vi "UDP Send (1).vi"(0 "Numeric 7":dbl, 1 "Numeric 3":dbl, 2 "Numeric 2":dbl, 3 "Numeric 4":dbl, 4 "Numeric 9":dbl, 5 "Numeric 8":dbl, 6 "Numeric":dbl, 7 "Numeric 5":dbl, 8 "Numeric 6":dbl) -> ()   [LabVIEW 2012]
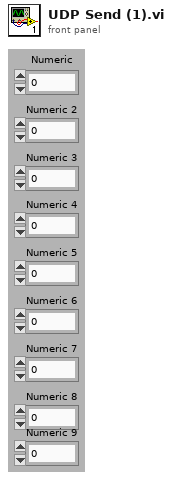
[diagram p1: front panel]
types:
  T1 = cluster{"Numeric":dbl, "Numeric 2":dbl, "Numeric 3":dbl, "Numeric 4":dbl, "Numeric 5":dbl, "Numeric 6":dbl, "Numeric 7":dbl, "Numeric 8":dbl, "Numeric 9":dbl}
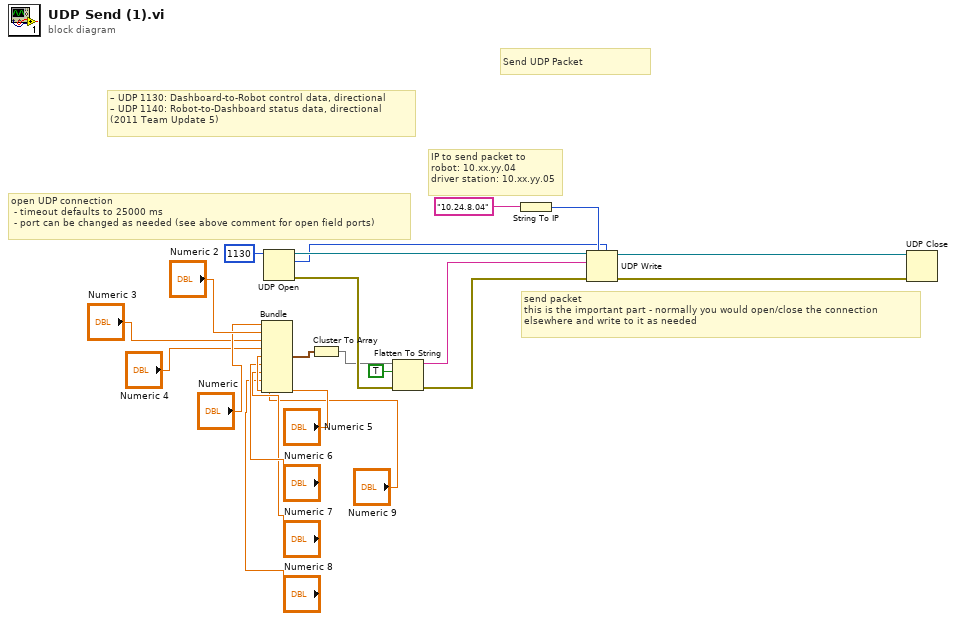
[diagram p0: block diagram]
diagram:
  # "send packet\nthis is the important part - normally you would open/close the connection \nelsewhere and write to it as needed"
  # "IP to send packet to \nrobot: 10.xx.yy.04\ndriver station: 10.xx.yy.05"
  # "open UDP connection\n - timeout defaults to 25000 ms\n - port can be changed as needed (see above comment for open field ports)"
  # "Send UDP Packet"
  # "– UDP 1130: Dashboard-to-Robot control data, directional\n– UDP 1140: Robot-to-Dashboard status data, directional\n(2011 Team Update 5)"
  n1 = Bundle("Numeric"="Numeric", "Numeric 2"="Numeric 2", "Numeric 3"="Numeric 3", "Numeric 4"="Numeric 4", "Numeric 5"="Numeric 5", "Numeric 6"="Numeric 6", "Numeric 7"="Numeric 7", "Numeric 8"="Numeric 8", "Numeric 9"="Numeric 9") -> (w3:T1)  [unwired: 1 in]
  n2 = UDP Open(11:u16 1130 ("port")) -> (port=w21:refnum<k16>, 0:w17:errorcluster, 2:w18:u16)  [unwired: 1 in, 3 out]
  n3 = Cluster To Array(cluster=w3) -> (array=w2:dbl[])
  n4 = Flatten To String(anything=w2, prepend array or string size? (T)=TRUE, error in (no error)=w17) -> (data string=w15:string, error out=w16:errorcluster)  [unwired: 2 out]
  n5 = String To IP(1:"10.24.8.04") -> (0:w19:u32)
  n6 = UDP Write(address=w19, port or service name=w18, connection ID=w21, data in=w15, 8:w16) -> (error out=w13:errorcluster, 3:w14:refnum<k16>)  [unwired: 1 out]
  n7 = UDP Close(connection ID=w14, 8:w13) -> ()  [unwired: 2 out]
